vi "Format CSV ONOFF.vi"(0 "Data_In":i32[](array[ring]) items=["OFF", "ON"]) -> (4 "Data_out":string)   [LabVIEW 2020, in "Anritsu Signal Analyzer Series.lvlib"]
doc: "Format ON/OFF Data to CSV Data String"
uses:
  Anritsu Signal Analyzer Series.lvlib
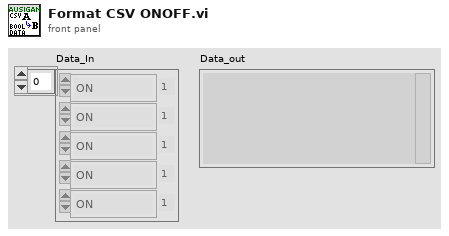
[diagram p1: front panel]
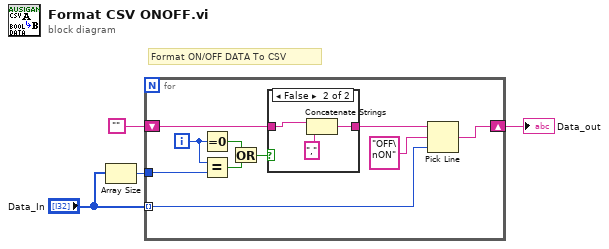
[diagram p0: block diagram]
diagram:
  # "Format ON/OFF DATA To CSV"
  n1 = Array Size(array="Data_In") -> (size(s)=w3:i32)
  n2 = for {
    tunnel: "Data_In" -> [w6] mode=indexing
    shift-right: [w5] -> w2
    shift-left: "" -> [w11]
    tunnel: w3 -> [w9]
    i -> [w10]
    n3 = Equal To 0?(x=w10) -> (x = 0?=w12:bool)
    n4 = Equal?(x=w10, y=w9) -> (x = y?=w13:bool)
    n5 = Or(x=w12, y=w13) -> (x .or. y?=w14:bool)
    n6 = case shown="False" w14 {
      tunnel: w11 -> [w15 w18]
      tunnel: [w15 w16] -> w7
      frame True {
      }
      frame False {
        n7 = Concatenate Strings(w18, "," ("string")) -> (w16:string)
      }
    }
    n8 = Pick Line(string ("")=w7, multi-line string="OFF\nON" ("複数行文字列"), line index=w6) -> (output string=w5:string)
  }
  "Data_out" <- w2
